vi "Identity Value.vi"(3 "Module Identity in":refnum<class "Module Identity.lvclass">) -> (1 "Value":string)   [LabVIEW 2020, in "Volatus.lvlib" / "Module Identity.lvclass"]
uses:
  Module Identity.lvclass
  Module Identity.lvclass/Module Identity.ctl
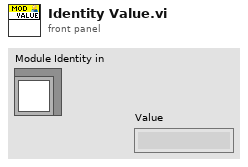
[diagram p1: front panel]
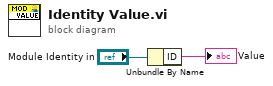
[diagram p0: block diagram]
diagram:
  n1 = Unbundle By Name("Module Identity in") -> ("ID"=→"Value":string)
